vi "(SubVI) Delete Noisy Force.vi"(4 "xDNA":dbl[](array[numeric]), 7 "Force":dbl[](array[numeric])) -> (0 "xDNA-cut":dbl[](array[numeric]), 3 "Force-cut":dbl[](array[numeric]))   [LabVIEW 2014]
panel:
  in  "xDNA lowercut":dbl
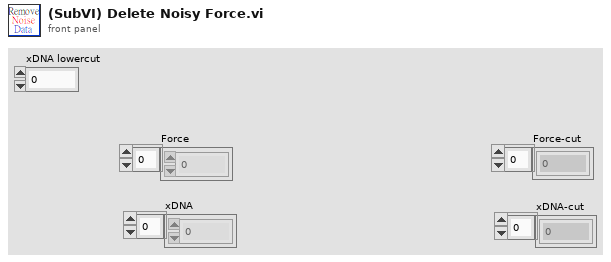
[diagram p1: front panel]
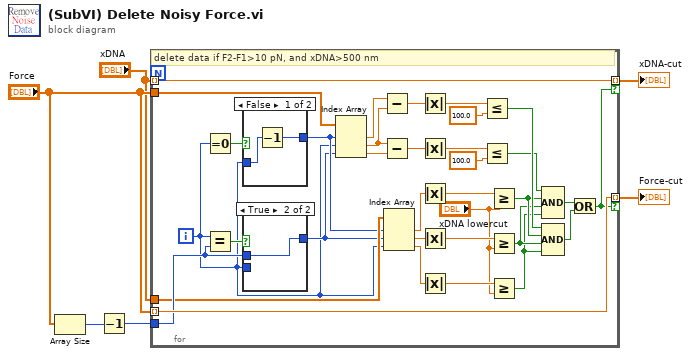
[diagram p0: block diagram]
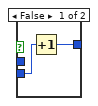
[diagram p2: hidden frame]
diagram:
  n1 = Array Size(array="Force") -> (size(s)=w3:i32)
  n2 = Decrement(x=w3) -> (x-1=w2:i32)
  n3 = for {
    tunnel: "xDNA" -> [w40] mode=indexing
    tunnel: "Force" -> [w39] mode=indexing
    tunnel: [w40] -> w6 mode=indexing if=w25
    tunnel: [w39] -> w5 mode=indexing if=w25
    tunnel: "Force" -> [w38]
    tunnel: w2 -> [w35]
    tunnel: "xDNA" -> [w24]
    i -> [w21]
    # "delete data if F2-F1>10 pN, and xDNA>500 nm"
    n4 = Equal To 0?(x=w21) -> (x = 0?=w37:bool)
    n5 = Equal?(x=w21, y=w35) -> (x = y?=w36:bool)
    n6 = case shown="False" w37 {
      tunnel: [w44 w46] -> w23
      tunnel: w21 -> [w45 w46]
      frame False {
        n7 = Decrement(x=w45) -> (x-1=w44:i32)
      }
      frame True {
      }
    }
    n8 = case shown="True" w36 {
      tunnel: [w41 w43] -> w22
      tunnel: w21 -> [w42 _]
      tunnel: w35 -> [_ w43]
      frame False {
        n9 = Increment(x=w42) -> (x+1=w41:i32)
      }
      frame True {
      }
    }
    n10 = Index Array(array=w38, index #1=w23, index #2=w21, index #3=w22) -> (element #1=w34:dbl, element #2=w33:dbl, element #3=w32:dbl)
    n11 = Subtract(x=w34, y=w33) -> (x-y=w30:dbl)
    n12 = Subtract(x=w33, y=w32) -> (x-y=w31:dbl)
    n13 = Index Array(array=w24, index #1=w23, index #2=w22, index #3=w21) -> (element #1=w13:dbl, element #2=w11:dbl, element #3=w9:dbl)
    n14 = Absolute Value(x=w30) -> (abs(x)=w29:dbl)
    n15 = Absolute Value(x=w31) -> (abs(x)=w26:dbl)
    n16 = Absolute Value(x=w13) -> (abs(x)=w12:dbl)
    n17 = Absolute Value(x=w11) -> (abs(x)=w10:dbl)
    n18 = Absolute Value(x=w9) -> (abs(x)=w8:dbl)
    n19 = Less Or Equal?(x=w29, y=100.0) -> (x <= y?=w20:bool)
    n20 = Less Or Equal?(x=w26, y=100.0) -> (x <= y?=w19:bool)
    n21 = Greater Or Equal?(x=w12, y="xDNA lowercut") -> (x >= y?=w18:bool)
    n22 = Greater Or Equal?(x=w10, y="xDNA lowercut") -> (x >= y?=w17:bool)
    n23 = Greater Or Equal?(x=w8, y="xDNA lowercut") -> (x >= y?=w16:bool)
    n24 = Compound Arithmetic op=AND(w19, w18, w17, w16) -> (w15:bool)
    n25 = Compound Arithmetic op=AND(w20, w18, w17, w16) -> (w14:bool)
    n26 = Or(x=w15, y=w14) -> (x .or. y?=w25:bool)
  }
  "xDNA-cut" <- w6
  "Force-cut" <- w5
